vi "Untitled 25 (SubVI).vi"(8 "error in (no error)":errorcluster, 11 "JKI SM in":refnum<class "JKI SM.lvclass">) -> (0 "error out":errorcluster, 3 "Class Name":string)   [LabVIEW 2013, in "JKI State Machine API.lvlib" / "JKI SM.lvclass"]
uses:
  JKI SM.lvclass
  JKI SM.lvclass/JKI SM.ctl
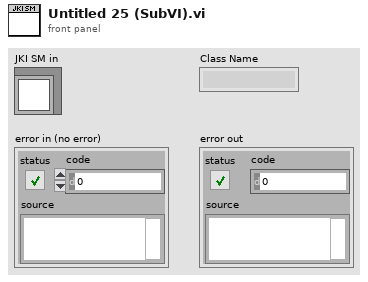
[diagram p1: front panel]
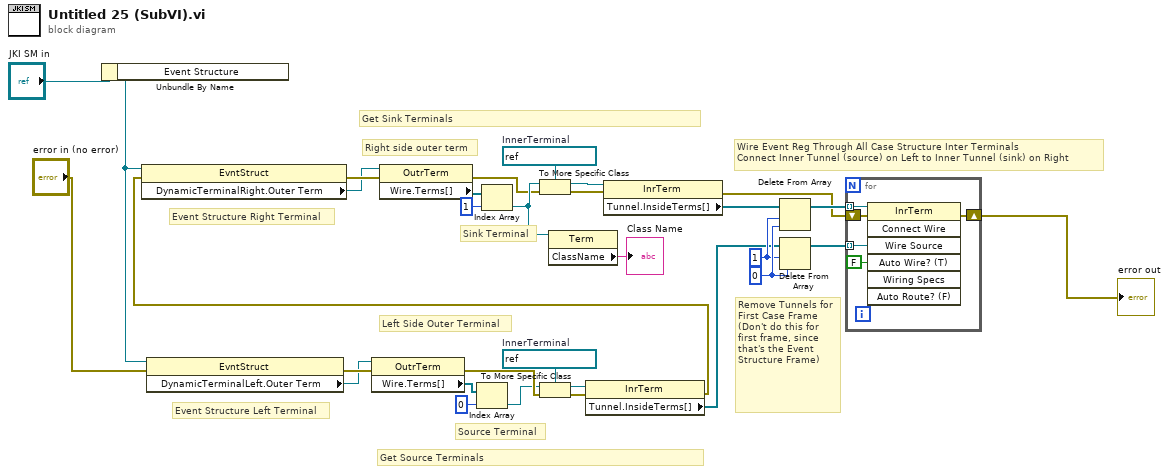
[diagram p0: block diagram]
diagram:
  w23 = 0 ("index")
  w22 = 1 ("length")
  w9 = refnum<vi> refnum  # InnerTerminal
  w3 = refnum<vi> refnum  # InnerTerminal
  # "Event Structure Right Terminal"
  # "Event Structure Left Terminal"
  # "Get Sink Terminals"
  # "Get Source Terminals"
  # "Remove Tunnels for First Case Frame\n(Don't do this for first frame, since that's the Event Structure Frame)"
  # "Wire Event Reg Through All Case Structure Inter Terminals\nConnect Inner Tunnel (source) on Left to Inner Tunnel (sink) on Right"
  # "Left Side Outer Terminal"
  # "Right side outer term"
  # "Source Terminal"
  # "Sink Terminal"
  n1 = Unbundle By Name("JKI SM in") -> ("Event Structure"=w29:refnum<vi>)
  n2 = property class="EvntStruct"(reference=w29, error in="error in (no error)") -> (error out=w31:errorcluster, "DynamicTerminalLeft.Outer Term"=w28:refnum<vi>)  [unwired: 1 out]
  n3 = property class="OutrTerm"(reference=w28, error in=w31) -> (error out=w16:errorcluster, "Wire.Terms[]"=w8:refnum<vi>[])  [unwired: 1 out]
  n4 = Index Array(array=w8, index=0) -> (element=w10:refnum<vi>)
  n5 = To More Specific Class(target class=w9, reference=w10, error in=w16) -> (specific class reference=w11:refnum<vi>, error out=w17:errorcluster)
  n6 = property class="InrTerm"(reference=w11, error in=w17) -> (error out=w26:errorcluster, "Tunnel.InsideTerms[]"=w18:refnum<vi>[])  [unwired: 1 out]
  n7 = property class="EvntStruct"(reference=w29, error in=w26) -> (error out=w27:errorcluster, "DynamicTerminalRight.Outer Term"=w25:refnum<vi>)  [unwired: 1 out]
  n8 = property class="OutrTerm"(reference=w25, error in=w27) -> (error out=w4:errorcluster, "Wire.Terms[]"=w1:refnum<vi>[])  [unwired: 1 out]
  n9 = Index Array(array=w1, index=1) -> (element=w13:refnum<vi>)
  n10 = To More Specific Class(target class=w3, reference=w13, error in=w4) -> (specific class reference=w5:refnum<vi>, error out=w6:errorcluster)
  n11 = property class="Term"(reference=w13) -> ("ClassName"=→"Class Name":string)  [unwired: 1 in, 2 out]
  n12 = property class="InrTerm"(reference=w5, error in=w6) -> (error out=w12:errorcluster, "Tunnel.InsideTerms[]"=w20:refnum<vi>[])  [unwired: 1 out]
  n13 = Delete From Array(array=w20, length=w22, index=w23) -> (array with subset deleted=w21:refnum<vi>[])  [unwired: 1 out]
  n14 = Delete From Array(array=w18, length=w22, index=w23) -> (array with subset deleted=w19:refnum<vi>[])  [unwired: 1 out]
  n15 = for {
    tunnel: w21 -> [w36] mode=indexing
    tunnel: w19 -> [w35] mode=indexing
    shift-right: [w33] -> w15
    shift-left: w12 -> [w32]
    n16 = invoke class="InrTerm" method="Connect Wire"(reference=w36, error in=w32, "Wire Source"=w35, "Auto Wire? (T)"=FALSE) -> (error out=w33:errorcluster)  [unwired: 3 in, 6 out]
  }
  "error out" <- w15
